vi "WPI_SonarSRF04DigitalRefNum Registry Set.vi"(8 "error in (no error)":errorcluster, 9 "Test Mode Only":bool, 10 "refnum name":string="My Sonar RefNum", 11 "SonarSRF04DevRef":T1={"DevStatus"={"status"=FALSE, "code"=0, "source"=""}, "Ping Channel"=enum."Invalid", "Echo Channel"=enum."Invalid", "CntIndex"=enum."Invalid"}) -> (0 "error out":errorcluster, 3 "SonarSRF04DevRef":T1={"DevStatus"={"status"=FALSE, "code"=0, "source"=""}, "Ping Channel"=enum."Invalid", "Echo Channel"=enum."Invalid", "CntIndex"=enum."Invalid"})   [LabVIEW 2017]
doc: "Sets a reference into a named registry storage. After setting a reference, you can retrieve it by name using the <B>RefNum Registry Get</B>.\nThe <B>Test Mode Only</B> parameter restricts it so Test Mode can use the reference, but other code cannot get the refnum and modify the I/O."
uses:
  <vilib>/Rock Robotics/WPI/Ultrasonic/WPI_UltrasonicDeviceRef.ctl
  <vilib>/Rock Robotics/SystemInterfaces/DIO/FPGA_DIOChannel.ctl
  <vilib>/Rock Robotics/SystemInterfaces/Counter/FPGA_CounterCtrSystemIndex.ctl
  <vilib>/Rock Robotics/WPI/Utilities/Refnum Registry Operation.ctl
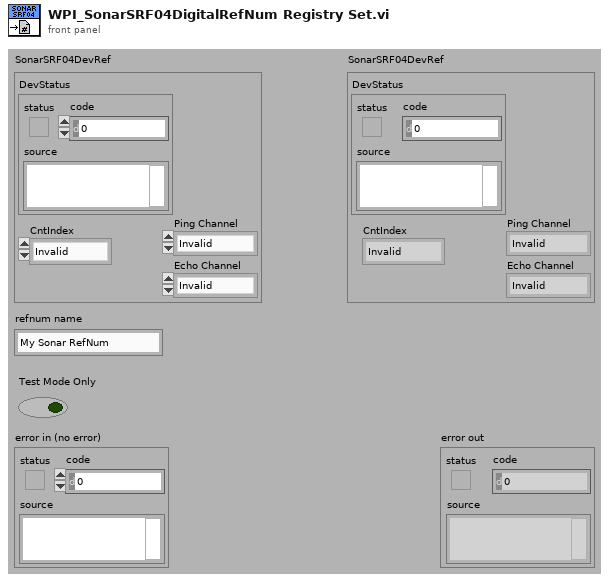
[diagram p1: front panel]
types:
  T1 = typedef "WPI_UltrasonicDeviceRef.ctl" = cluster{"DevStatus":errorcluster, "Ping Channel":T2, "Echo Channel":T2, "CntIndex":T3}
  T2 = typedef "FPGA_DIOChannel.ctl" = enum8{"DIO 0", "DIO 1", "DIO 2", "DIO 3", "DIO 4", "DIO 5", "DIO 6", "DIO 7", "DIO 8", "DIO 9", "DIO MXP 0", "DIO MXP 1", "DIO MXP 2", "DIO MXP 3", "DIO MXP 4", "DIO MXP 5", "DIO MXP 6", "DIO MXP 7", "DIO MXP 8", "DIO MXP 9", "DIO MXP 10", "DIO MXP 11", "DIO MXP 12", "DIO MXP 13", "DIO MXP 14", "DIO MXP 15", "SPI Port CS1", "SPI Port CS2", "SPI Port CS3", "SPI Port MISO", "SPI Port MOSI", "Invalid"}
  T3 = typedef "FPGA_CounterCtrSystemIndex.ctl" = enum8{"Ctr 0", "Ctr 1", "Ctr 2", "Ctr 3", "Ctr 4", "Ctr 5", "Ctr 6", "Ctr 7", "Invalid"}
  T4 = typedef "Refnum Registry Operation.ctl" = enum16{"set", "get", "delete", "get all names", "read name"}
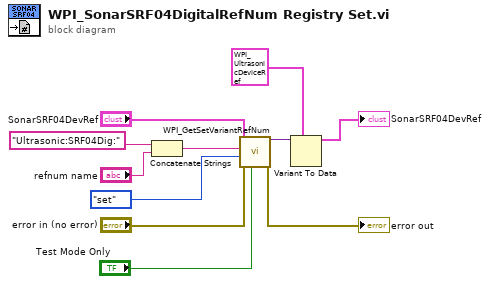
[diagram p0: block diagram]
diagram:
  n1 = Concatenate Strings("Ultrasonic:SRF04Dig:", "refnum name") -> (w11:string)
  n2 = call <vilib>:"WPI_GetSetVariantRefNum.vi"("Test Mode Only"="Test Mode Only", "error in (no error)"="error in (no error)", "Operation"=Refnum_Registry_Operation."set" ("menu"), "refnum name"=w11, "DevRef"="SonarSRF04DevRef") -> ("error out"=→"error out":errorcluster, "DevRef"=w9:variant)  [unwired: 4 in, 1 out]
  n3 = Variant To Data(type=T1 {"DevStatus"={"status"=FALSE, "code"=0, "source"=""}, "Ping Channel"=enum."Invalid", "Echo Channel"=enum."Invalid", "CntIndex"=enum."Invalid"} ("SonarSRF04DevRef"), Variant=w9) -> (data=→"SonarSRF04DevRef":T1)  [unwired: 1 in, 1 out]
